vi "U16 Shifter by 2.vi"(4 "Shift":u8, 6 "Flush Data":bool, 8 "Input Valid":bool, 11 "Current Data":u32 format="%.0x") -> (0 "Output Data Valid":bool, 3 "Shifted Data":u32 format="%.0x")   [LabVIEW 2011]
doc: "This VI combines data from two consecutive samples based on shifter position. This is useful when combining data from parallel streams based on trigger position."
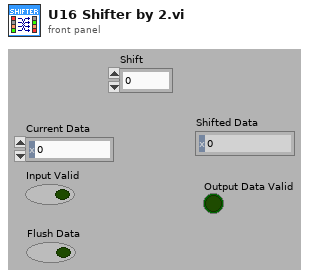
[diagram p1: front panel]
types:
  T1 = cluster{"Previous Data":u32, "Previous Data Valid":bool}
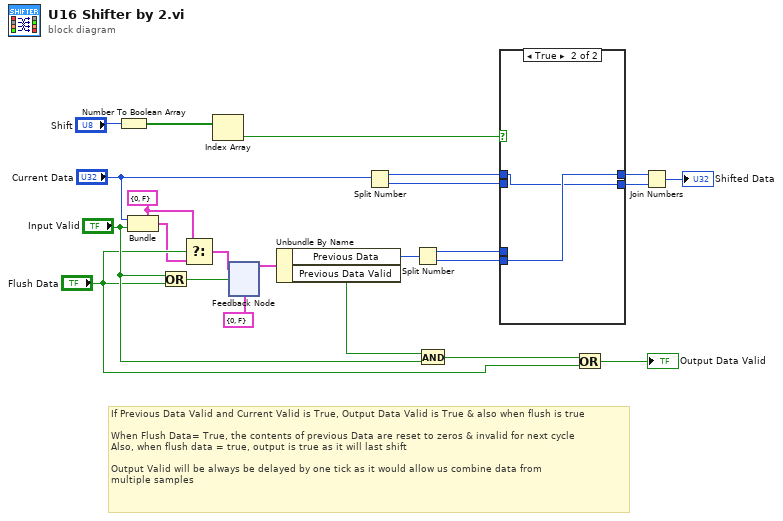
[diagram p0: block diagram]
diagram:
  w1 = T1 {"Previous Data"=0, "Previous Data Valid"=FALSE} ("cluster")
  # "If Previous Data Valid and Current Valid is True, Output Data Valid is True & also when flush is true\n\nWhen Flush Data= True, the contents of previous Data are reset to zeros & invalid for next cycle\nAlso, when flush data = true, output is true as it will last shift\n\nOutput Valid will be always be delayed by one tick as it would allow us combine data from\nmultiple samples"
  n1 = Number To Boolean Array(number="Shift") -> (Boolean array=w21:bool[])
  n2 = Bundle(cluster=w1, "Previous Data"="Current Data", "Previous Data Valid"="Input Valid") -> (w2:T1)
  n3 = Or(x="Input Valid", y="Flush Data") -> (x .or. y?=w9:bool)
  n4 = Select(t=w1, s="Flush Data", f=w2) -> (s? t:f=w4:T1)
  n5 = Index Array(array=w21) -> (element=w22:bool)  [unwired: 1 in]
  n6 = feedback-in #1(w4, w9) -> ()
  n7 = feedback #1(T1 {"Previous Data"=0, "Previous Data Valid"=FALSE} ("cluster")) -> (w12:T1)
  n8 = Unbundle By Name(w12) -> ("Previous Data"=w11:u32, "Previous Data Valid"=w10:bool)
  n9 = Split Number(x="Current Data") -> (hi(x)=w20:u16, lo(x)=w19:u16)
  n10 = Split Number(x=w11) -> (hi(x)=w18:u16, lo(x)=w17:u16)
  n11 = And(x=w10, y="Input Valid") -> (x .and. y?=w7:bool)
  n12 = case shown="True" w22 {
    tunnel: w20 -> [_ w26]
    tunnel: w19 -> [_ _]
    tunnel: w18 -> [w25 _]
    tunnel: w17 -> [w24 w27]
    tunnel: [w25 w27] -> w16
    tunnel: [w24 w26] -> w15
    frame False {
    }
    frame True {
    }
  }
  n13 = Or(x=w7, y="Flush Data") -> (x .or. y?=→"Output Data Valid":bool)
  n14 = Join Numbers(hi=w16, lo=w15) -> ((hi.lo)=→"Shifted Data":u32)
